vi "vscan.vi"(0 "IP adress":string="192.109.209.229", 1 "stop":bool, 2 "Channel":u8(ring) items=["1", "2", "3", "4", "5", "6", "7", "8", "9", "10", "11", "12", "13", "14", "15", "16"], 3 "VSCAN Parameters":T1={"tb"=5e-05, "vs_initial "=TRUE, "Voltage_step"=0.0, "Scans"=[{" vs_initial "=FALSE, "Voltage_step"=0.1, "Scan_Rate"=0.1}, {" vs_initial "=FALSE, "Voltage_step"=-0.2, "Scan_Rate"=0.1}, {" vs_initial "=FALSE, "Voltage_step"=0.0, "Scan_Rate"=0.1}], "Scan_number"=2, "N_Cycles"=0, "Record_every_dE"=0.01, "Begin_measuring_I"=0.5, "End_measuring_I"=0.75, "I_Range"=12, "E_Range"=3, "Bandwidth"=5, "em"=1, "ce"=0} {"tb" min=5e-05 max=1 format="%^_3e"; "ce" items=["Standard", "CE to ground"]; "End_measuring_I" min=0 max=1 format="%.2f"; "Begin_measuring_I" min=0 max=1 format="%.2f"; "Voltage_step" min=-10 max=10 format="%^_3e"; "N_Cycles" min=0 max=1000000; "Scan_number" min=0 max=98; "Scans"."Scan_Rate" min=1e-05 max=10 format="%^_3e"; "Scans"."Voltage_step" format="%^_3e"; "E_Range" items=["±2.5V", "±5V", "±10V", "Auto"]; "Bandwidth" items=["1"=1, "2"=2, "3"=3, "4"=4, "5"=5, "6"=6, "7"=7, "8"=8, "9"=9]; "Record_every_dE" format="%^_3e"; "I_Range" items=["1pA", "1nA", "10nA", "100nA", "1µA", "10µA", "100µA", "1mA", "10mA", "100mA", "1A", "Booster", "Auto"]}, 4 "Exit":bool, 5 "Start":bool, 6 "Draw":enum16{"I(Ewe)", "Ewe(t)", "I(t)"}(ring)=enum."Ewe(t)") -> (7 "XY Graph":cluster{"Data 101":sgl[], "Data 101":sgl[]}(graph)={"Data 101"=[8e-05, 0.1006, 0.20111999, 0.30164, 0.40219998, 0.50272, 0.60324, 0.70375997, 0.80428, 0.90484, 1.002, 1.10252, 1.20304, 1.30356, 1.40412, 1.50464, 1.60516, 1.70568, 1.8061999, 1.90676, 2.0072799, 2.1078, 2.20832, 2.3088799, 2.4094, 2.50992, 2.61044, 2.711, 2.8115199, 2.91204, 3.01256, 3.1131198, 3.21364, 3.3141599, 3.41468, 3.5152, 3.6157598, 3.71628, 3.8167999, 3.91732, 4.00108, 4.1015997, 4.20212, 4.30264, 4.4031997, 4.50372, 4.60424, 4.70476, 4.8052797, 4.90584, 5.00636, 5.1068797, 5.2074, 5.30796, 5.4084797, 5.509, 5.60952, 5.7100797, 5.8106, 5.91112], "Data 101"=[4.2835555e-07, 2.1494968e-06, 4.146294e-06, 6.138965e-06, 8.133681e-06, 1.0123058e-05, 1.2087297e-05, 1.4083101e-05, 1.6065378e-05, 1.80591e-05, 1.9984154e-05, 1.7937375e-05, 1.595267e-05, 1.3964497e-05, 1.197563e-05, 9.982255e-06, 7.9902675e-06, 6.0027883e-06, 3.9787647e-06, 1.9855738e-06, -3.2822256e-09, -1.9828094e-06, -3.9722895e-06, -5.9632257e-06, -7.95541e-06, -9.9489125e-06, -1.1902557e-05, -1.389385e-05, -1.5878555e-05, -1.7874703e-05, -1.9867039e-05, -2.1852784e-05, -2.3842693e-05, -2.583641e-05, -2.7823196e-05, -2.9813451e-05, -3.180405e-05, -3.3791526e-05, -3.5780395e-05, -3.777169e-05, -3.9435956e-05, -3.7391255e-05, -3.539476e-05, -3.3405893e-05, -3.1415642e-05, -2.9424347e-05, -2.7433402e-05, -2.5453895e-05, -2.3455323e-05, -2.1465068e-05, -1.9473428e-05, -1.7484906e-05, -1.5494306e-05, -1.3505094e-05, -1.1516228e-05, -9.523894e-06, -7.5357216e-06, -5.542347e-06, -3.5301439e-06, -1.543508e-06]}, 8 "Number of points":i32=60)   [LabVIEW 2015]
doc: "The VSCAN ( Potentiodynamic Technique) consists of scanning linearly the potential of a stationary working electrode with different scan rates.\nIn general, in this VI, the first thing to do is to start by establishing the connection with the instrument defined by its IP adress, then load the firmware in the channel selected, get the information on the plugged channels, load protocol on a channel, start/stop the protocol, retreive data and draw the graph."
uses:
  base_xml.llb/Type Descriptor Enumeration__ogtk.ctl
panel:
  out "Device Code":i32=12
  out "Exit 2":bool=TRUE
  out "Data 124":sgl[][](array[numeric])=[[8e-05, -0.00015008324, 4.2835555e-07, 0.0013634439, 1.0], [0.1006, 0.009902848, 2.1494968e-06, 0.010471455, 1.0], [0.20111999, 0.019955778, 4.146294e-06, 0.02059764, 1.0], [0.30164, 0.030008709, 6.138965e-06, 0.030609425, 1.0], [0.40219998, 0.04006164, 8.133681e-06, 0.04071481, 1.0], [0.50272, 0.050114572, 1.0123058e-05, 0.05077513, 1.0], [0.60324, 0.060167503, 1.2087297e-05, 0.06075918, 1.0], [0.70375997, 0.07022043, 1.4083101e-05, 0.07082297, 1.0], [0.80428, 0.08027337, 1.6065378e-05, 0.080852084, 1.0], [0.90484, 0.090326294, 1.80591e-05, 0.090902, 1.0], [1.002, 0.10004413, 1.9984154e-05, 0.100629516, 1.0], [1.10252, 0.0899912, 1.7937375e-05, 0.09124173, 1.0], [1.20304, 0.07993827, 1.595267e-05, 0.08120915, 1.0], [1.30356, 0.069885336, 1.3964497e-05, 0.0711627, 1.0], [1.40412, 0.059832405, 1.197563e-05, 0.06106771, 1.0], [1.50464, 0.049779475, 9.982255e-06, 0.051007397, 1.0], [1.60516, 0.039726544, 7.9902675e-06, 0.040967878, 1.0], [1.70568, 0.029673612, 6.0027883e-06, 0.030924892, 1.0], [1.8061999, 0.019620681, 3.9787647e-06, 0.020868042, 1.0], [1.90676, 0.009567751, 1.9855738e-06, 0.010804256, 1.0], [2.0072799, -0.00048518094, -3.2822256e-09, 0.0006746042, 1.0], [2.1078, -0.010538111, -1.9828094e-06, -0.009257445, 1.0], [2.20832, -0.020591041, -3.9722895e-06, -0.019307364, 1.0], [2.3088799, -0.030643972, -5.9632257e-06, -0.029412746, 1.0], [2.4094, -0.0406969, -7.95541e-06, -0.039452266, 1.0], [2.50992, -0.050749835, -9.9489125e-06, -0.049533386, 1.0], [2.61044, -0.060802765, -1.1902557e-05, -0.059479296, 1.0], [2.711, -0.07085569, -1.389385e-05, -0.06955695, 1.0], [2.8115199, -0.08090863, -1.5878555e-05, -0.07963461, 1.0], [2.91204, -0.09096155, -1.7874703e-05, -0.08969492, 1.0], [3.01256, -0.10101449, -1.9867039e-05, -0.09973444, 1.0], [3.1131198, -0.111067414, -2.1852784e-05, -0.1098225, 1.0], [3.21364, -0.12112035, -2.3842693e-05, -0.119851604, 1.0], [3.3141599, -0.13117327, -2.583641e-05, -0.12988071, 1.0], [3.41468, -0.1412262, -2.7823196e-05, -0.13995838, 1.0], [3.5152, -0.15127914, -2.9813451e-05, -0.15000136, 1.0], [3.6157598, -0.16133207, -3.180405e-05, -0.16006514, 1.0], [3.71628, -0.17138499, -3.3791526e-05, -0.1701324, 1.0], [3.8167999, -0.18143792, -3.5780395e-05, -0.18019964, 1.0], [3.91732, -0.19149086, -3.777169e-05, -0.19023915, 1.0], [4.00108, -0.1998683, -3.9435956e-05, -0.19861813, 1.0], [4.1015997, -0.18981537, -3.7391255e-05, -0.1892373, 1.0], [4.20212, -0.17976244, -3.539476e-05, -0.17914924, 1.0], [4.30264, -0.1697095, -3.3405893e-05, -0.16911319, 1.0], [4.4031997, -0.15965658, -3.1415642e-05, -0.15908061, 1.0], [4.50372, -0.14960365, -2.9424347e-05, -0.14899254, 1.0], [4.60424, -0.13955072, -2.7433402e-05, -0.13895303, 1.0], [4.70476, -0.12949778, -2.5453895e-05, -0.12891698, 1.0], [4.8052797, -0.119444855, -2.3455323e-05, -0.11883587, 1.0], [4.90584, -0.10939193, -2.1465068e-05, -0.10876862, 1.0], [5.00636, -0.09933899, -1.9473428e-05, -0.098690964, 1.0], [5.1068797, -0.08928607, -1.7484906e-05, -0.088686116, 1.0], [5.2074, -0.07923313, -1.5494306e-05, -0.07859806, 1.0], [5.30796, -0.069180205, -1.3505094e-05, -0.06854121, 1.0], [5.4084797, -0.059127275, -1.1516228e-05, -0.05848783, 1.0], [5.509, -0.049074344, -9.523894e-06, -0.048455246, 1.0], [5.60952, -0.039021414, -7.5357216e-06, -0.038367193, 1.0], [5.7100797, -0.028968483, -5.542347e-06, -0.028327677, 1.0], [5.8106, -0.018915553, -3.5301439e-06, -0.018236158, 1.0], [5.91112, -0.008862623, -1.543508e-06, -0.008182773, 1.0]] format="%.2f"
  # "Instructions:\nBefore running the VI you must type a valid IP adress that corresponds to the instrument.Then press the Run button to execute this VI.\nWhile this VI is running, choose the available channel, enter the VSCAN parameters or keep the default values, then press the button start to begin the experience.\nChoose the waveform to draw (Ewe(t) or I(t) or I(Ewe) or Ec(t). You can stop the measure if you press the stop button and exit the execution if you press the exit button."
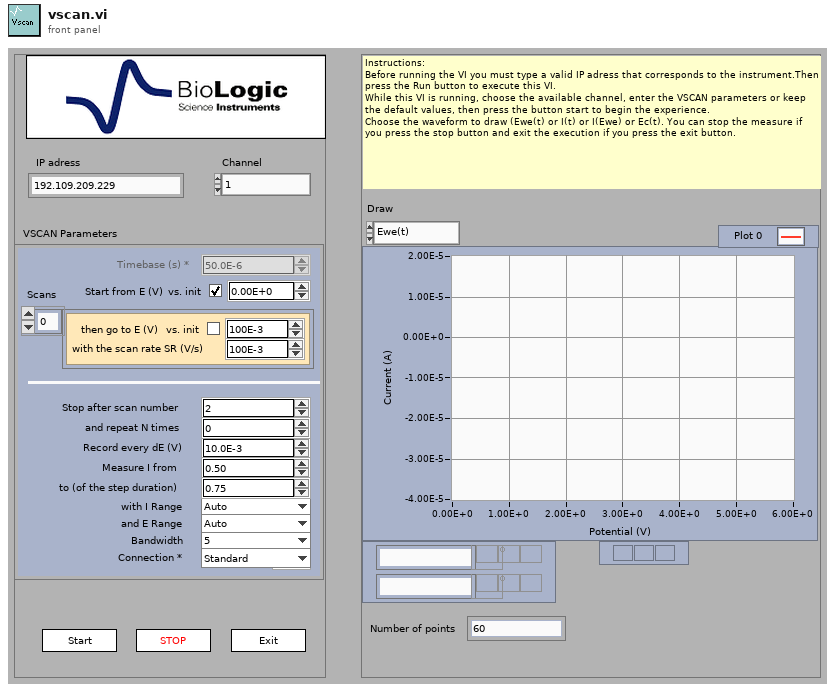
[diagram p1: front panel]
types:
  T1 = cluster{"tb":sgl, "vs_initial ":bool, "Voltage_step":sgl, "Scans":cluster{" vs_initial ":bool, "Voltage_step":sgl, "Scan_Rate":sgl}[], "Scan_number":i32, "N_Cycles":i32, "Record_every_dE":sgl, "Begin_measuring_I":sgl, "End_measuring_I":sgl, "I_Range":u16, "E_Range":u16, "Bandwidth":u16, "em":u16, "ce":u16}
  T2 = typedef "Type Descriptor Enumeration__ogtk.ctl" = enum8{"<Null>", "I8", "I16", "I32", "I64", "U8", "U16", "U32", "U64", "SGL", "DBL", "EXT", "CSG", "CDB", "CXT", "0x0F", "0x10", "0x11", "0x12", "0x13", "0x14", "Enum U8", "Enum U16", "Enum U32", "Enum U64", "SGL PQ", "DBL PQ", "EXT PQ", "CSG PQ", "CDB PQ", "CXT PQ", "0x1F", "0x20", "Boolean", "0x22", "0x23", "0x24", "0x25", "0x26", "0x27", "0x28", "0x29", "0x2A", "0x2B", "0x2C", "0x2D", "0x2E", "0x2F", "String", "0x31", "Path", "Pict", "0x34", "0x35", "0x36", "DAQ", "0x38", "0x39", "0x3A", "0x3B", "0x3C", "0x3D", "0x3E", "0x3F", "Array", "0x41", "0x42", "0x43", "0x44", "0x45", "0x46", "0x47", "0x48", "0x49", "0x4A", "0x4B", "0x4C", "0x4D", "0x4E", "0x4F", "Cluster", "0x51", "0x52", "Variant", "Waveform", "0x55", "0x56", "0x57", "0x58", "0x59", "0x5A", "0x5B", "0x5C", "0x5D", "0x5E", "0x5F", "0x60", "0x61", "0x62", "0x63", "0x64", "0x65", "0x66", "0x67", "0x68", "0x69", "0x6A", "0x6B", "0x6C", "0x6D", "0x6E", "0x6F", "Refnum"}
  T3 = cluster{"Data Type":T2, "Format String":string}[]
  T4 = cluster{"Channel":i32, "BoardVersion":i32, "BoardSerialCode":i32, "FirmwareCode":i32, "FirmwareVersion":i32, "XilinxVersion":i32, "AmpCode":i32, "NbAmp":i32, "LcBoard":i32, "Zboard":i32, "MuxBoard":i32, "GPRAboard":i32, "MemSize":i32, "MemFilled":i32, "state":i32, "MaxIRange":i32, "MinIRange":i32, "MaxBandwidth":i32, "NbOfTechniques":i32}
  T5 = cluster{" vs_initial ":bool, "Voltage_step":sgl, "Scan_Rate":sgl}[]
  T6 = cluster{" vs_initial ":bool, "Voltage_step":sgl, "Scan_Rate":sgl}
  T7 = cluster{"Label":string, "type":i32, "valeur":u32, "index":i32}[]
  T8 = cluster{"IRQskipped":i32, "NbRaws":i32, "NbCols":i32, "Technique Index":i32, "TechniqueID":i32, "PrcessIndex":i32, "loop":i32, "StartTime":dbl, "MuxPad":i32}
  T9 = cluster{"State":i32, "MemFilled":i32, "TimeBase":sgl, " Ewe":sgl, " EweRangeMin":sgl, " EweRangeMax":sgl, "Ece":sgl, "EceRangeMin":sgl, "EceRangeMax":sgl, "Eoverflow":i32, "I":sgl, "IRange":i32, "Ioverflow":i32, "ElapsedTime":sgl, "Freq":sgl, "Rcomp":sgl, "Saturation":sgl, "OptErr":i32, "OptPos":i32}
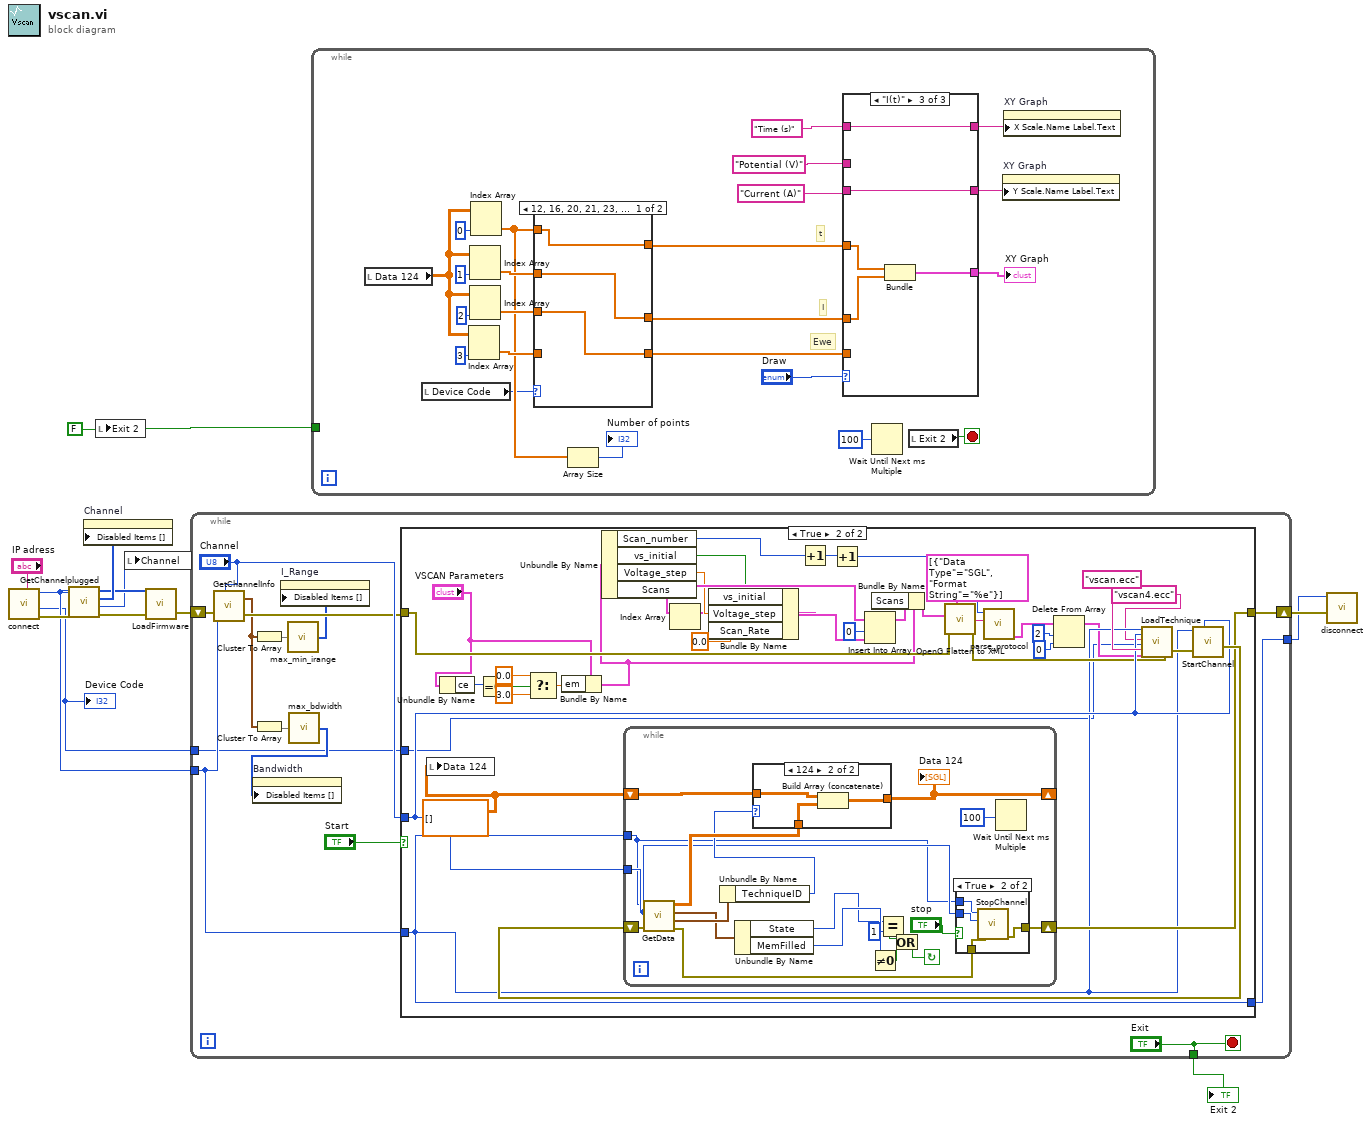
[diagram p0: block diagram]
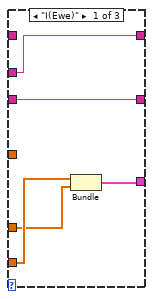
[diagram p2: hidden frame]
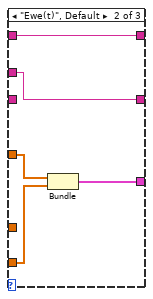
[diagram p3: hidden frame]
diagram:
  w12 = FALSE ("Exit 2")
  n1 = call "connect.vi"("IP"="IP adress") -> ("error out"=w10:errorcluster, "Device Code"=w1:i32, "ID"=w3:i32)  [unwired: 7 in, 1 out]
  "Device Code" <- w1
  n2 = call "GetChannelplugged.vi"("error in (no error)"=w10, "ID"=w3) -> ("error out"=w7:errorcluster, "First channel"=w5:i32, "Disabled channels"=w9:i32[], "Plugged channels"=w8:i32[])  [unwired: 6 in]
  n3 = property on="Channel" class="Ring (strict)"("Disabled Items []"=w9) -> ()  [unwired: 2 in, 2 out]
  n4 = local write "Exit 2"(w12) -> ()
  n5 = local write "Channel"(w5) -> ()
  n6 = call "LoadFirmware.vi"("error in (no error)"=w7, "Channels"=w8, "ID"=w3) -> ("error out"=w4:errorcluster)  [unwired: 7 in, 1 out]
  n7 = while {
    shift-right: [w26] -> w11
    shift-left: w4 -> [w23]
    tunnel: ["Exit"] -> w13
    tunnel: w3 -> [w16]
    tunnel: [w15] -> w2
    tunnel: w1 -> [w14]
    stop <- "Exit" stop-if-true
    n8 = call "GetChannelInfo.vi"("error in (no error)"=w23, "Channel"="Channel", "ID"=w16) -> ("error out"=w22:errorcluster, "Channel information"=w19:T4)  [unwired: 7 in]
    n9 = Cluster To Array(cluster=w19) -> (array=w21:i32[])
    n10 = Cluster To Array(cluster=w19) -> (array=w20:i32[])
    n11 = call "max_min_irange.vi"("resources"=w21) -> ("disabled ranges"=w17:i32[])
    n12 = property on="I_Range" class="Ring (strict)"("Disabled Items []"=w17) -> ()  [unwired: 2 in, 2 out]
    n13 = call "max_bdwidth.vi"("resources"=w20) -> ("disabled ranges"=w18:i32[])
    n14 = property on="Bandwidth" class="Ring (strict)"("Disabled Items []"=w18) -> ()  [unwired: 2 in, 2 out]
    n15 = case shown="True" "Start" {
      tunnel: "Channel" -> [_ w60]
      tunnel: [w29 w62] -> w26
      tunnel: w22 -> [w29 w57]
      tunnel: w16 -> [w28 w55]
      tunnel: [w28 w55] -> w15
      tunnel: w14 -> [_ w30]
      frame False {
      }
      frame True {
        w61 = sgl[][] []
        n16 = local write "Data 124"(w61) -> ()
        n17 = Unbundle By Name("VSCAN Parameters") -> ("ce"=w35:u16)
        n18 = Equal To 0?(x=w35) -> (x = 0?=w34:bool)
        n19 = Select(t=0.0, s=w34, f=3.0) -> (s? t:f=w37:dbl)
        n20 = Bundle By Name(cluster="VSCAN Parameters", "em"=w37) -> (w32:T1)
        n21 = Unbundle By Name(w32) -> ("Scan_number"=w40:i32, "vs_initial"=w45:bool, "Voltage_step"=w46:sgl, "Scans"=w49:T5)
        n22 = Index Array(array=w49) -> (element=w43:T6)  [unwired: 1 in]
        n23 = Bundle By Name(cluster=w43, "vs_initial"=w45, "Voltage_step"=w46, "Scan_Rate"=sgl 0.0) -> (w47:T6)
        n24 = Increment(x=w40) -> (x+1=w41:i32)
        n25 = Increment(x=w41) -> (x+1=w39:i32)
        n26 = Insert Into Array(array=w49, index=0 ("indice"), new element=w47) -> (w50:T5)
        n27 = Bundle By Name(cluster=w32, "Scans"=w50) -> (w42:T1)
        n28 = call "OpenG Flatten to XML.vi"("Type Formats (default)"=T3 [{"Data Type"=enum."SGL", "Format String"="%e"}] ("Type Formats"), "error in (no error)"=w57, "LabVIEW Data"=w42) -> ("error out"=w56:errorcluster, "XML String"=w58:string)  [unwired: 7 in]
        n29 = call "parse_protocol.vi"("XML String In"=w58, "index array"=w39) -> ("Params Values"=w52:T7)  [unwired: 7 in]
        n30 = Delete From Array(array=w52, length=2 ("longueur"), index=0 ("indice")) -> (array with subset deleted=w51:T7)  [unwired: 1 out]
        n31 = call "LoadTechnique.vi"("ID"=w55, "Selected Channel"=w60, "FName4"="vscan4.ecc" ("FName"), "Device Code"=w30, "FName"="vscan.ecc", "Protocol Parameters"=w51, "error in (no error)"=w56) -> ("error out"=w64:errorcluster)  [unwired: 12 in]
        n32 = call "StartChannel.vi"("error in (no error)"=w64, "Channel"=w60, "ID"=w55) -> ("error out"=w63:errorcluster)  [unwired: 8 in]
        n33 = while {
          shift-right: [w77] -> w62
          shift-left: w63 -> [w80]
          shift-right: [w74] -> _
          shift-left: w61 -> [w75]
          tunnel: w60 -> [w70]
          tunnel: w55 -> [w69]
          stop <- w78 continue-if-true
          n34 = call "GetData.vi"("error in (no error)"=w80, "Channel"=w70, "ID"=w69) -> ("error out"=w73:errorcluster, "Data information"=w84:T8, "Current values"=w68:T9, "Data"=w76:dbl[][])  [unwired: 5 in]
          n35 = Unbundle By Name(w84) -> ("TechniqueID"=w72:i32)
          n36 = Unbundle By Name(w68) -> ("State"=w66:i32, "MemFilled"=w67:i32)
          n37 = case shown="124" w72 {
            tunnel: w76 -> [_ w93]
            tunnel: w75 -> [w90 w92]
            tunnel: [w90 w91] -> w74
            frame 0, Default {
            }
            frame 124 {
              n38 = Build Array (concatenate)(w92, w93) -> (w91:dbl[][])
            }
          }
          "Data 124" <- w74
          n39 = Not Equal To 0?(x=w67) -> (x != 0?=w81:bool)
          n40 = Equal?(x=w66, y=1) -> (x = y?=w82:bool)
          n41 = Or(x=w82, y=w81) -> (x .or. y?=w78:bool)
          n42 = case shown="True" "stop" {
            tunnel: [w85 w89] -> w77
            tunnel: w73 -> [w85 w88]
            tunnel: w70 -> [_ w87]
            tunnel: w69 -> [_ w86]
            frame False {
            }
            frame True {
              n43 = call "StopChannel.vi"("error in (no error)"=w88, "Channel"=w87, "ID"=w86) -> ("error out"=w89:errorcluster)  [unwired: 8 in]
            }
          }
          n44 = Wait Until Next ms Multiple(millisecond multiple=u32 100) -> ()  [unwired: 1 out]
        }
      }
    }
  }
  "Exit 2" <- w13
  n45 = while {
    tunnel: w12 -> [_]
    stop <- w115 stop-if-true
    # "Ewe"
    # "I"
    # "t"
    n46 = local read "Data 124"() -> (w106:sgl[][])
    n47 = local read "Device Code"() -> (w104:i32)
    n48 = Index Array(array=w106, index (col)=3 ("Index")) -> (element=w108:sgl[])  [unwired: 1 in]
    n49 = Index Array(array=w106, index (col)=1 ("Index")) -> (element=w111:sgl[])  [unwired: 1 in]
    n50 = Index Array(array=w106, index (col)=2 ("Index")) -> (element=w109:sgl[])  [unwired: 1 in]
    n51 = Index Array(array=w106, index (col)=0 ("Index")) -> (element=w105:sgl[])  [unwired: 1 in]
    n52 = case shown="12, 16, 20, 21, 23, 27" w104 {
      tunnel: w111 -> [w133 _]
      tunnel: w109 -> [w132 w136]
      tunnel: w108 -> [_ w135]
      tunnel: w105 -> [w134 w137]
      tunnel: [w134 w137] -> w96
      tunnel: [w133 w136] -> w95
      tunnel: [w132 w135] -> w94
      frame 12, 16, 20, 21, 23, 27 {
      }
      frame Default {
      }
    }
    n53 = Array Size(array=w105) -> (size(s)=→"Number of points":i32)
    n54 = case shown="\"I(t)\"" "Draw" {
      tunnel: w96 -> [_ w126 w131]
      tunnel: w95 -> [w118 _ w130]
      tunnel: [w117 w122 w127] -> w103
      tunnel: "Potential (V)" ("Y Scale.Name Label.Text") -> [w121 w125 _]
      tunnel: "Current (A)" ("Y Scale.Name Label.Text") -> [w120 _ w129]
      tunnel: [w120 w125 w129] -> w101
      tunnel: [w121 w124 w128] -> w100
      tunnel: "Time (s)" ("Y Scale.Name Label.Text") -> [_ w124 w128]
      tunnel: w94 -> [w119 w123 _]
      frame "I(Ewe)" {
        n55 = Bundle("Data 124"=w119, "Data 124"=w118) -> (w117:cluster{"Data 124":sgl[], "Data 124":sgl[]})  [unwired: 1 in]
      }
      frame "Ewe(t)", Default {
        n56 = Bundle("Data 124"=w126, "Data 124"=w123) -> (w122:cluster{"Data 124":sgl[], "Data 124":sgl[]})  [unwired: 1 in]
      }
      frame "I(t)" {
        n57 = Bundle("Data 124"=w131, "Data 124"=w130) -> (w127:cluster{"Data 124":sgl[], "Data 124":sgl[]})  [unwired: 1 in]
      }
    }
    "XY Graph" <- w103
    n58 = Wait Until Next ms Multiple(millisecond multiple=u32 100) -> ()  [unwired: 1 out]
    n59 = local read "Exit 2"() -> (w115:bool)
    n60 = property on="XY Graph" class="XYGraph (strict)"("Y Scale.Name Label.Text"=w101) -> ()  [unwired: 2 in, 2 out]
    n61 = property on="XY Graph" class="XYGraph (strict)"("X Scale.Name Label.Text"=w100) -> ()  [unwired: 2 in, 2 out]
  }
  n62 = call "disconnect.vi"("error in (no error)"=w11, "ID"=w2) -> ()  [unwired: 9 in, 1 out]
